vi "Update Sub Export.vi"(0 "NSIS_Installer in":refnum<class "Compound_Installer.lvclass">, 5 "Sub Export":refnum<class "Export.lvclass">, 11 "error in (no error)":errorcluster) -> (4 "NSIS_Installer out":refnum<class "Compound_Installer.lvclass">, 15 "error out":errorcluster)   [LabVIEW 2017, in "CL_G3_VIComponentBuilder.lvlib" / "Compound_Installer.lvclass"]
doc: "Updates the sub export by unique name in the sub installers lookup table."
uses:
  Compound_Installer.lvclass
  Exports/Export.lvclass
  Compound_Installer.lvclass/Compound_Installer.ctl
  Exports/Export.lvclass/Export.ctl
  Exports/Accessors/Read unique Name.vi
  Accessors/Read Sub Exports.vi
  Accessors/Write Sub Exports.vi
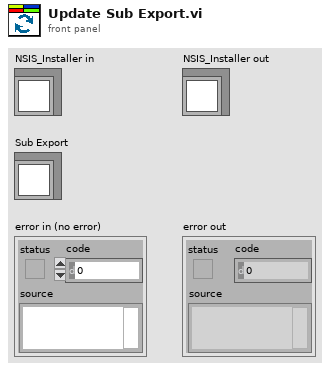
[diagram p1: front panel]
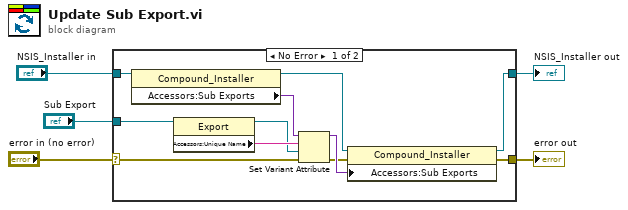
[diagram p0: block diagram]
diagram:
  n1 = case shown="No Error" "error in (no error)" {
    selector: "error in (no error)" -> [w6 w18]
    tunnel: [w7 w18] -> w4
    tunnel: [w9 w17] -> w2
    tunnel: "NSIS_Installer in" -> [w10 w17]
    tunnel: "Sub Export" -> [w8 _]
    frame No Error {
      n2 = property class="Compound_Installer"(reference=w10) -> (reference out=w16:refnum<class "Compound_Installer.lvclass">, "Accessors:Sub Exports"=w15:variant)  [unwired: 1 in, 1 out]
      n3 = property class="Export"(reference=w8) -> (reference out=w12:refnum<class "Export.lvclass">, "Accessors:Unique Name"=w13:string)  [unwired: 1 in, 1 out]
      n4 = Set Variant Attribute(Variant=w15, name=w13, value=w12, error in=w6) -> (Variant out=w14:variant, error out=w11:errorcluster)  [unwired: 1 out]
      n5 = property class="Compound_Installer"(reference=w16, error in=w11, "Accessors:Sub Exports"=w14) -> (reference out=w9:refnum<class "Compound_Installer.lvclass">, error out=w7:errorcluster)
    }
    frame Error {
    }
  }
  "error out" <- w4
  "NSIS_Installer out" <- w2
